vi "SystemParameters.vi"() -> ()   [LabVIEW 2013]
panel:
  in  "System Parameters":T1={"defaultLanguage"="fr", "languageFile"="lang.csv", "languages"="en;fr;de;es", "calibrationVolumeFile"="CalibrationVolumeFile.dat", "machineName"=""}
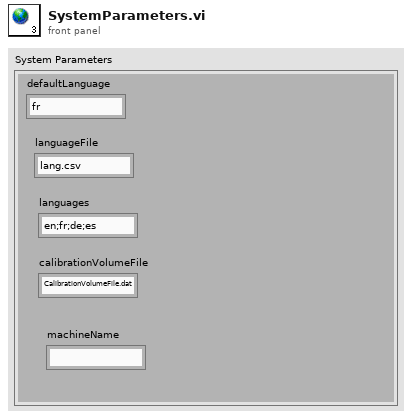
[diagram p1: front panel]
types:
  T1 = cluster{"defaultLanguage":string, "languageFile":string, "languages":string, "calibrationVolumeFile":string, "machineName":string}
diagram:
